vi "Copy sxp comments to de-embedded file.vi"(5 "Filename has to include:":string="p_DUT", 7 "Standalone":bool=TRUE, 11 "SnP File Path":path) -> ()   [LabVIEW 2020]
panel:
  out "Files copied":i32
  in  "Play":bool
  in  "Location":enum16{"Beginning", "End"}(ring)
  out "Horizontal Progress Bar":u8(slide) scale=0.0..100.0
  out "Status":string
  in  "Exit":bool
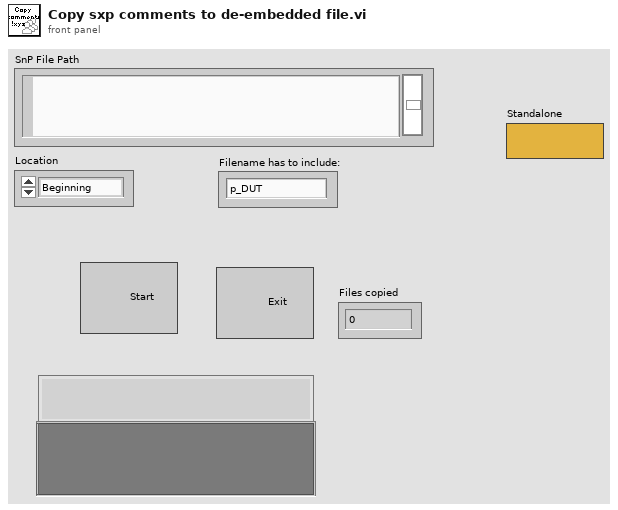
[diagram p1: front panel]
types:
  T1 = enum8{"Enabled", "Disabled", "Disabled and Grayed Out"}
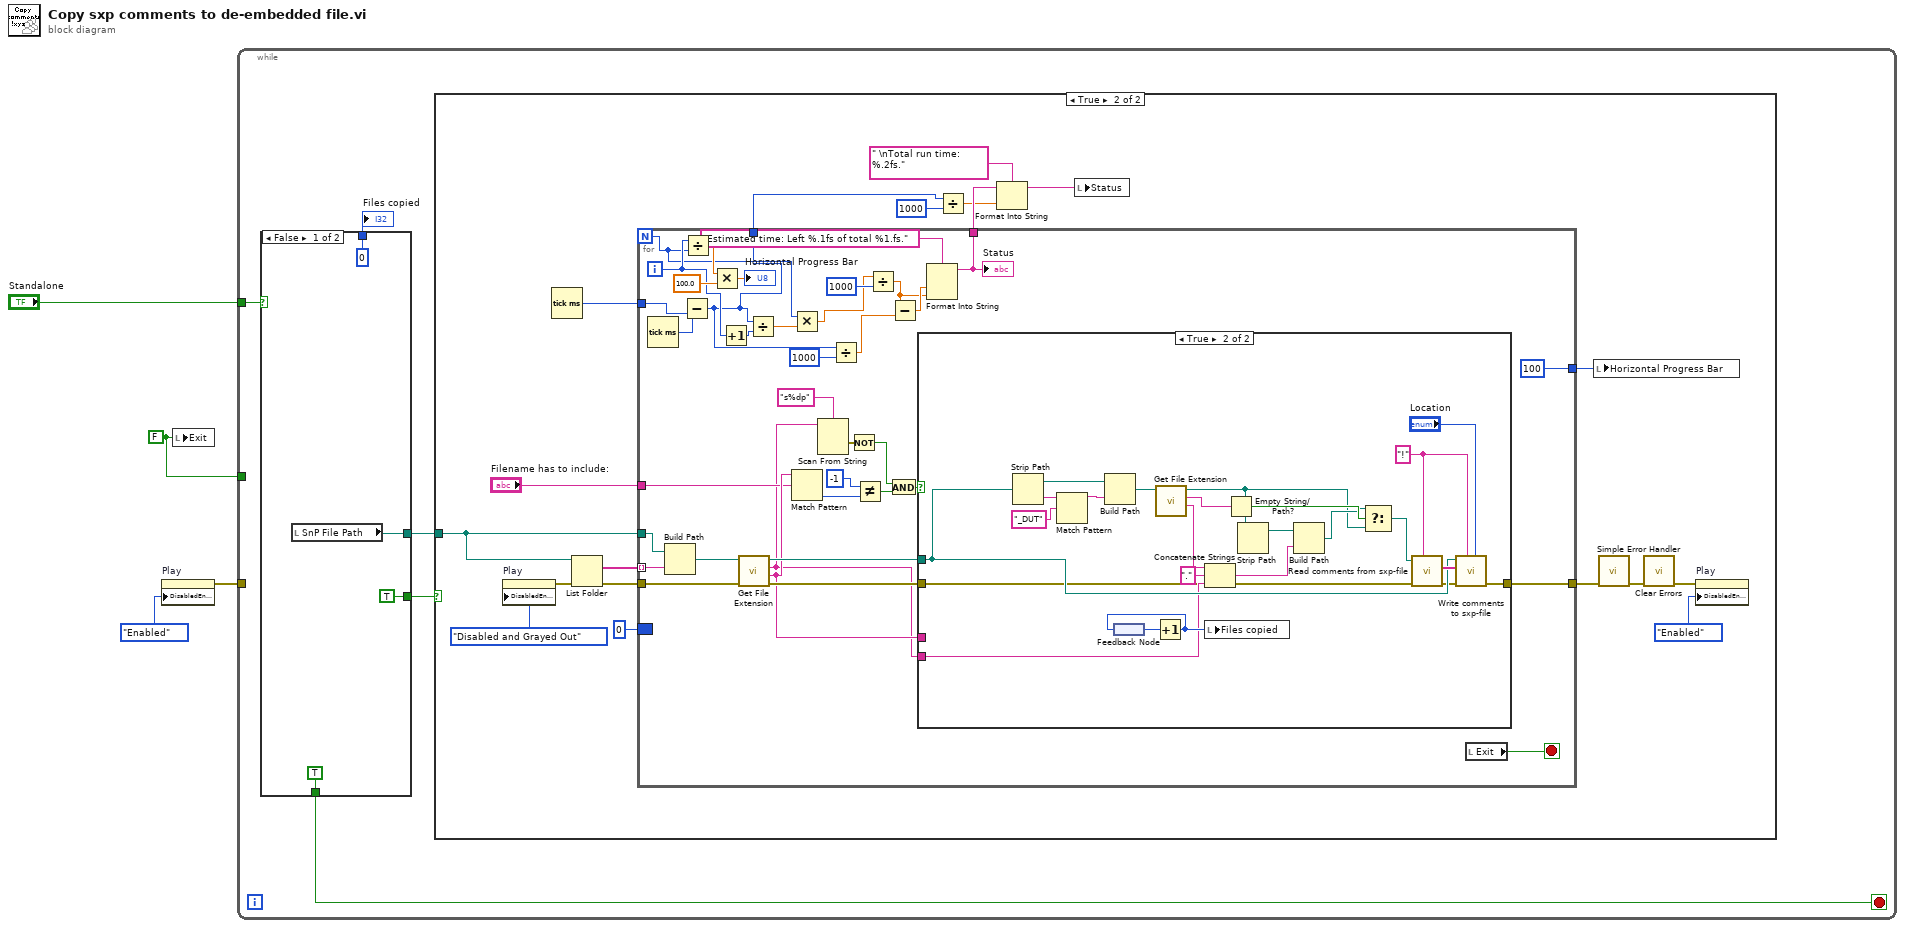
[diagram p0: block diagram]
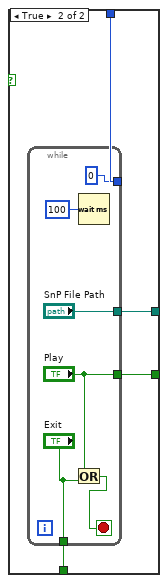
[diagram p2: hidden frame]
diagram:
  w2 = FALSE ("Exit")
  n1 = property on="Play" class="Bool"("DisabledEnum"=T1."Enabled" ("Disabled")) -> (error out=w3:errorcluster)  [unwired: 2 in, 1 out]
  n2 = local write "Exit"(w2) -> ()
  n3 = while {
    tunnel: w3 -> [_]
    tunnel: w2 -> [_]
    tunnel: "Standalone" -> [w5]
    stop <- w8 stop-if-true
    n4 = case shown="False" w5 {
      tunnel: [TRUE ("Play") w17] -> w9
      tunnel: [TRUE ("Exit") w16] -> w8
      tunnel: [0 ("y") w15] -> w7
      tunnel: [w13 w14] -> w6
      frame False {
        n5 = local read "SnP File Path"() -> (w13:path)
      }
      frame True {
        n6 = while {
          tunnel: ["Play"] -> w17
          tunnel: ["Exit"] -> w16
          tunnel: [0 ("y")] -> w15
          tunnel: ["SnP File Path"] -> w14
          stop <- w23 stop-if-true
          n7 = Or(x="Play", y="Exit") -> (x .or. y?=w23:bool)
          n8 = Wait (ms)(milliseconds to wait=u32 100) -> ()  [unwired: 1 out]
        }
      }
    }
    "Files copied" <- w7
    n9 = case shown="True" w9 {
      tunnel: w6 -> [_ w27]
      frame False {
      }
      frame True {
        n10 = property on="Play" class="Bool"("DisabledEnum"=T1."Disabled and Grayed Out" ("Disabled")) -> (error out=w37:errorcluster)  [unwired: 2 in, 1 out]
        n11 = Tick Count (ms)() -> (millisecond timer value=w34:u32)
        n12 = List Folder(path=w27, error in=w37) -> (filenames=w42:string[], error out=w41:errorcluster)  [unwired: 2 in, 2 out]
        n13 = for {
          N -> [w57]
          tunnel: w27 -> [w71]
          tunnel: [w79] -> w26
          tunnel: w41 -> [w75]
          tunnel: w42 -> [w47] mode=indexing
          tunnel: "Filename has to include:" -> [w68]
          tunnel: [u8 100 ("Horizontal Progress Bar")] -> w40
          tunnel: w34 -> [w62]
          tunnel: [w49] -> w32
          tunnel: [w48] -> w31
          border: 0 -> [_]
          i -> [w60]
          stop <- w63 stop-if-true
          n14 = Tick Count (ms)() -> (millisecond timer value=w61:u32)
          n15 = Build Path(base path=w71, name or relative path=w47) -> (appended path=w73:path)
          n16 = Subtract(x=w61, y=w62) -> (x-y=w49:u32)
          n17 = Divide(x=w60, y=w57) -> (x/y=w67:dbl)
          n18 = Multiply(x=w67, y=100.0) -> (x*y=→"Horizontal Progress Bar":dbl)
          n19 = Increment(x=w60) -> (x+1=w59:i32)
          n20 = call <vilib>:"Get File Extension.vi"("error in (no error)"=w75, "file"=w73) -> ("error out"=w74:errorcluster, "filename without extension"=w69:string, "lowercase file extension"=w43:string, "dup file"=w70:path)  [unwired: 5 in, 1 out]
          n21 = Divide(x=w49, y=w59) -> (x/y=w58:dbl)
          n22 = Multiply(x=w57, y=w58) -> (x*y=w51:dbl)
          n23 = Match Pattern(string=w69, regular expression=w68) -> (offset past match=w72:i32)  [unwired: 1 in, 3 out]
          n24 = Scan From String(format string="s%dp", input string=w43) -> (error out=w45:errorcluster)  [unwired: 4 in, 2 out]
          n25 = Divide(x=w49, y=u32 1000) -> (x/y=w54:dbl)
          n26 = Not(x=w45) -> (.not. x?=w44:bool)
          n27 = Not Equal?(x=-1, y=w72) -> (x != y?=w78:bool)
          n28 = Divide(x=w51, y=u32 1000) -> (x/y=w50:dbl)
          n29 = And(x=w44, y=w78) -> (x .and. y?=w76:bool)
          n30 = Subtract(x=w50, y=w54) -> (x-y=w53:dbl)
          n31 = case shown="True" w76 {
            tunnel: w70 -> [_ w99]
            tunnel: [w80 w97] -> w79
            tunnel: w74 -> [w80 w81]
            tunnel: w69 -> [_ _]
            tunnel: w43 -> [_ w88]
            frame False {
            }
            frame True {
              w94 = "!" ("Comment character")
              n32 = Strip Path(path=w99) -> (stripped path=w101:path, name=w104:string)
              n33 = Match Pattern(string=w104, regular expression="_DUT" ("Filename has to include:")) -> (before substring=w102:string)  [unwired: 1 in, 3 out]
              n34 = Build Path(base path=w101, name or relative path=w102) -> (appended path=w93:path)
              n35 = feedback #1() -> (w96:i32)
              n36 = Increment(x=w96) -> (x+1=w95:i32)
              n37 = feedback-in #1(w95) -> ()
              n38 = call <vilib>:"Get File Extension.vi"("file"=w93) -> ("filename without extension"=w90:string, "lowercase file extension"=w92:string, "dup file"=w84:path)  [unwired: 6 in, 2 out]
              n39 = Concatenate Strings(w90, "." ("string"), w88) -> (w87:string)
              n40 = local write "Files copied"(w95) -> ()
              n41 = Empty String/Path?(string/path=w92) -> (empty?=w86:bool)
              n42 = Strip Path(path=w84) -> (stripped path=w91:path)  [unwired: 1 out]
              n43 = Build Path(base path=w91, name or relative path=w87) -> (appended path=w85:path)
              n44 = Select(t=w85, s=w86, f=w84) -> (s? t:f=w83:path)
              n45 = call "Read comments from sxp-file.vi"("Comment character"=w94, "error in (no error)"=w81, "file path"=w83) -> ("error out"=w82:errorcluster, "Comment lines"=w100:string[])  [unwired: 6 in, 1 out]
              n46 = call "Write comments to sxp-file.vi"("Location"="Location", "Comment character"=w94, "error in (no error)"=w82, "Comment lines"=w100, "file path"=w99) -> ("error out"=w97:errorcluster)  [unwired: 5 in, 1 out]
            }
          }
          n47 = Format Into String(format string="Estimated time: Left %.1fs of total %1.fs.", w53, w50) -> (resulting string=w48:string)  [unwired: 2 in, 1 out]
          "Status" <- w48
          n48 = local read "Exit"() -> (w63:bool)
        }
        n49 = Divide(x=w32, y=u32 1000) -> (x/y=w28:dbl)
        n50 = Format Into String(format string=" \nTotal run time: %.2fs.", initial string=w31, w28) -> (resulting string=w30:string)  [unwired: 1 in, 1 out]
        n51 = local write "Status"(w30) -> ()
        n52 = local write "Horizontal Progress Bar"(w40) -> ()
        n53 = call <vilib>:"Simple Error Handler.vi"("error in (no error)"=w26) -> ("error out"=w36:errorcluster)  [unwired: 4 in, 4 out]
        n54 = call <vilib>:"Clear Errors.vi"("error in (no error)"=w36) -> ("error out"=w35:errorcluster)  [unwired: 5 in, 1 out]
        n55 = property on="Play" class="Bool"(error in=w35, "DisabledEnum"=T1."Enabled" ("Disabled")) -> ()  [unwired: 1 in, 2 out]
      }
    }
  }
